vi "[GV]_GPS Port NUM.vi"() -> ()   [LabVIEW 2016]
panel:
  in  "GPS port in":refnum<visa-resource-name>="COM9"
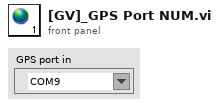
[diagram p1: front panel]
diagram:
